vi "traj_generator.vi"(0 "v_max":dbl, 1 "a_max":dbl, 2 "p_i":dbl, 3 "p_f":dbl, 4 "v_i":dbl, 5 "v_f":dbl, 6 "trigger":bool, 7 "t":dbl) -> (14 "p":dbl format="%0.2f", 15 "v":dbl format="%0.2f", 16 "a":dbl)   [LabVIEW 2012]
doc: "Based on :\nTime-Optimal Online Trajectory Generator for Robotic Manipulators \nFransisco Ramos. et al.\n\nInputs:\na_max = maximum admissible acceleration\nv_max = maximum admissible speed\np_i = current position\np_f = target position\nv_i = current velocity\nv_f = target velocity\ntrigger = tell the algorithm to proceed\nThe trigger signal is a transition from 0 to 1 (edge triggered)\n\nOutputs:\na = acceleration trajectory\nv = velocitiy trajectory\np = position trajectory"
panel:
  out "is_triggered":bool
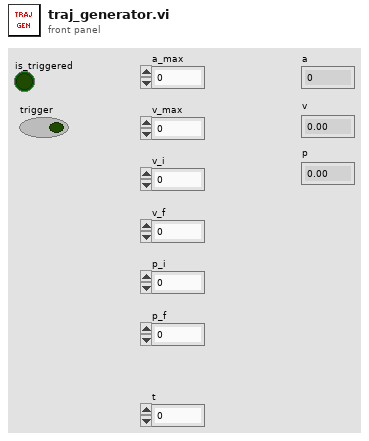
[diagram p1: front panel]
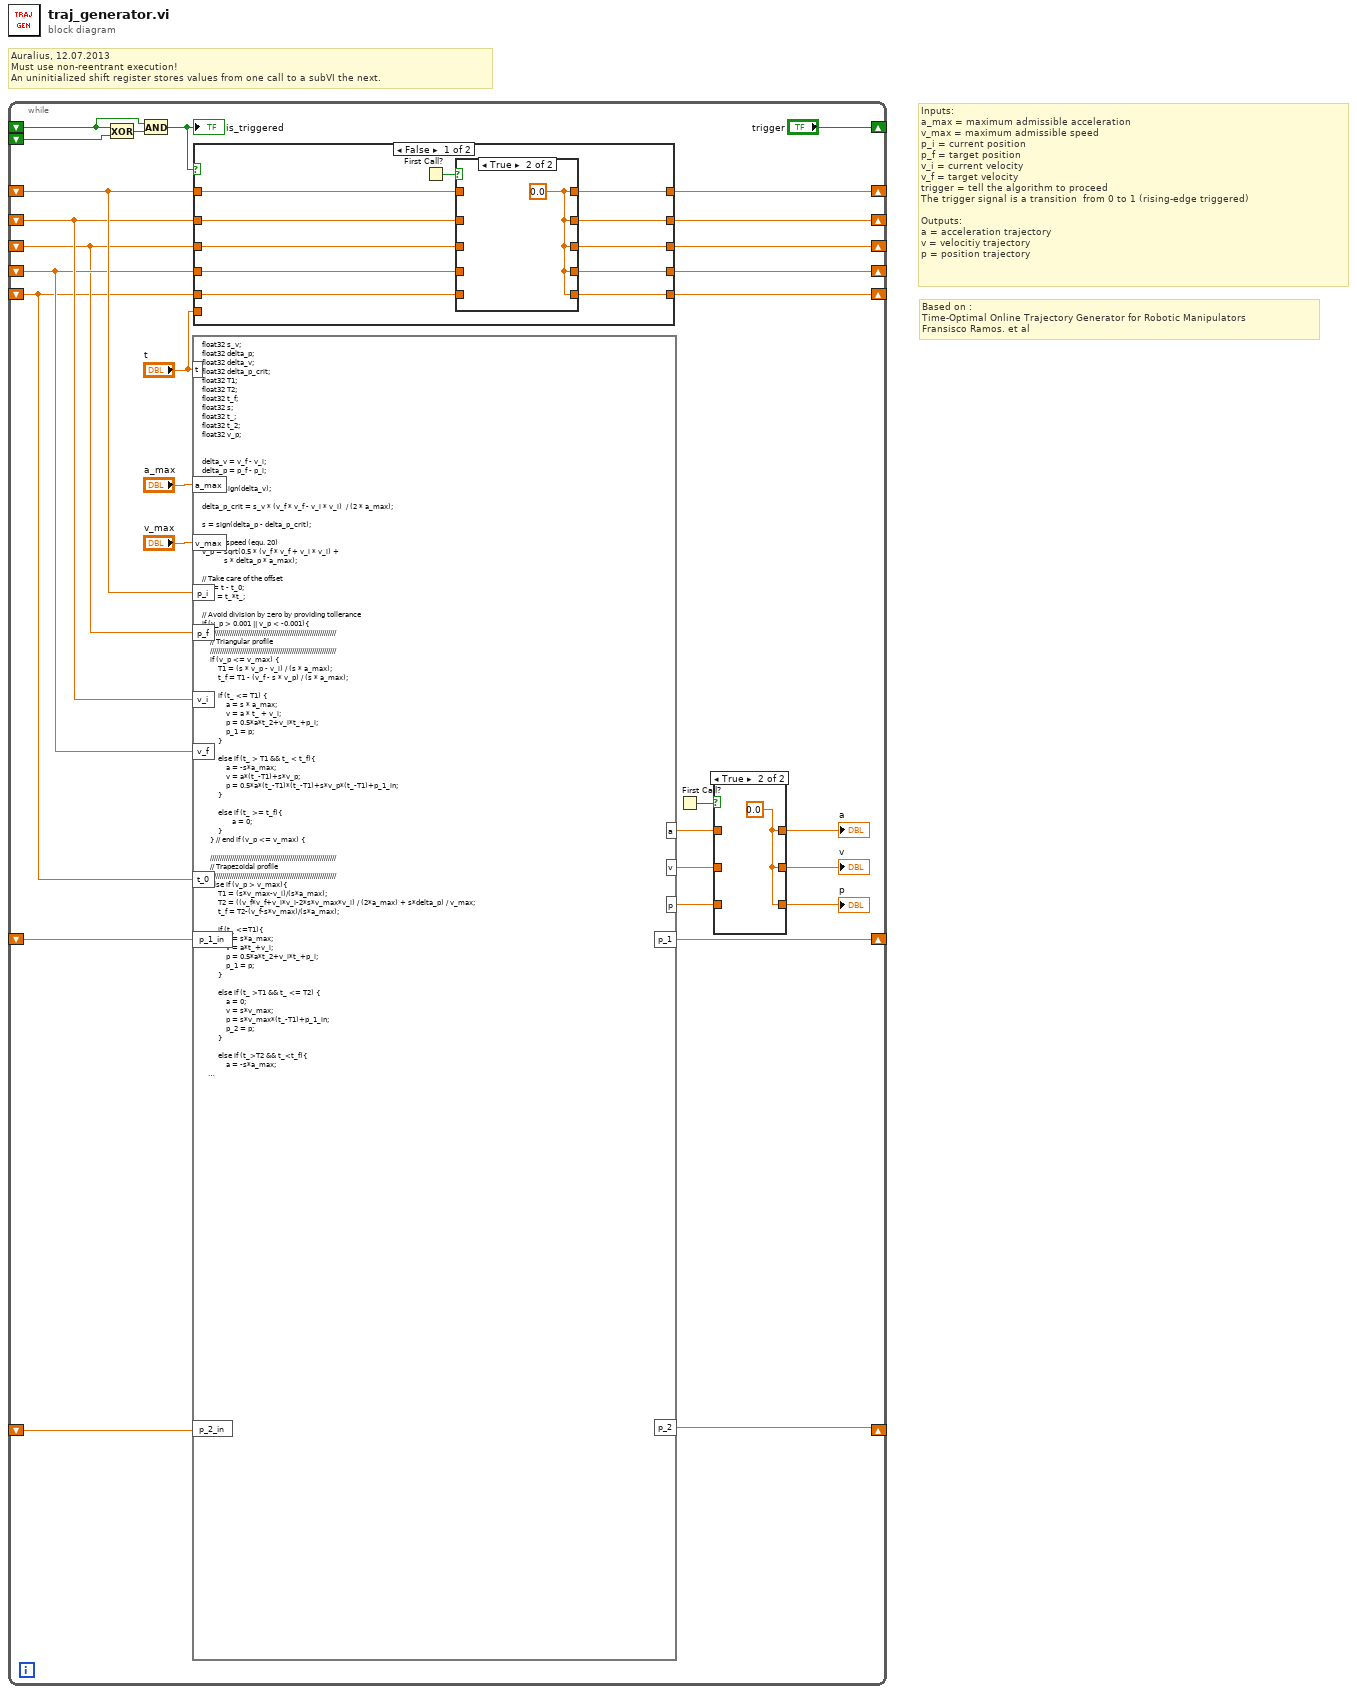
[diagram p0: block diagram]
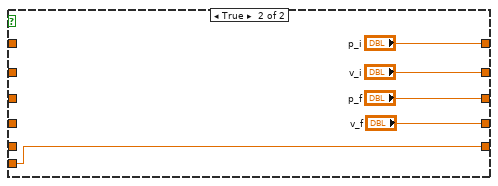
[diagram p4: hidden frame]
diagram:
  # "Based on :\nTime-Optimal Online Trajectory Generator for Robotic Manipulators \nFransisco Ramos. et al"
  # "Inputs:\na_max = maximum admissible acceleration\nv_max = maximum admissible speed\np_i = current position\np_f = target position\nv_i = current velocity\nv_f = target velocity\ntrigger = tell the algorithm to proceed\nThe trigger signal is a transition  from 0 to 1 (rising-edge triggered)\n\nOutputs:\na = acceleration trajectory\nv = velocitiy trajectory\np = position trajectory"
  # "Auralius, 12.07.2013\nMust use non-reentrant execution!\nAn uninitialized shift register stores values from one call to a subVI the next."
  n1 = while {
    shift-right: ["trigger"] -> _
    shift-left: _ -> [w25]
    shift-left: _ -> [w26]
    shift-right: [w23] -> _
    shift-left: _ -> [w21]
    shift-right: [w22] -> _
    shift-left: _ -> [w20]
    shift-right: [w18] -> _
    shift-left: _ -> [w15]
    shift-right: [w17] -> _
    shift-left: _ -> [w16]
    shift-right: [w14] -> _
    shift-left: _ -> [w13]
    shift-right: [w9] -> _
    shift-left: _ -> [w10]
    shift-right: [w8] -> _
    shift-left: _ -> [w7]
    stop <- FALSE continue-if-true
    n2 = Exclusive Or(1:w26, 2:w25) -> (0:w24:bool)
    n3 = And(x=w25, y=w24) -> (x .and. y?=w1:bool)
    "is_triggered" <- w1
    n4 = formula code="float32 s_v;\nfloat32 delta_p;\nfloat32 delta_v;\nfloat32 delta_p_crit;\nfloat32 T1;\nfloat32 T2;\nfloat32 t_f;\nfloat32 s;\nfloat32 t_;\nfloat32 t_2;\nfloat32 v_p;\n\n\ndelta_v = v_f - v_i;\ndelta_p = p_f - p_i;\n\ns_v = sign(delta_v);\n\ndelta_p_crit = s_v * (v_f * v_f - v_i * v_i)  / (2 * a_max);\n\ns = sign(delta_p - delta_p_crit);\n\n// Peak speed (equ. 20)\nv_p = sqrt(0.5 * (v_f * v_f + v_i * v_i) + \n           s * delta_p * a_max);\n\n// Take care of the offset\n t_ = t - t_0;\n t_2 = t_*t_;\n\n// Avoid division by zero by providing tollerance          \nif (v_p > 0.001 || v_p < -0.001){\n    ///////////////////////////////////////////////////////////////\n    // Triangular profile\n    ///////////////////////////////////////////////////////////////\n    if (v_p <= v_max) {\n        T1 = (s * v_p - v_i) / (s * a_max);\n        t_f = T1 - (v_f - s * v_p) / (s * a_max);\n\n        if (t_ <= T1) {\n            a = s * a_max;\n            v = a * t_ + v_i;\n            p = 0.5*a*t_2+v_i*t_+p_i;\n            p_1 = p;\n        } \n\n        else if (t_ > T1 && t_ < t_f){\n            a = -s*a_max;\n            v = a*(t_-T1)+s*v_p;\n            p = 0.5*a*(t_-T1)*(t_-T1)+s*v_p*(t_-T1)+p_1_in;\n        }\n\n        else if (t_ >= t_f){\n               a = 0;\n        }\n    } // end if (v_p <= v_max) {\n\n    ///////////////////////////////////////////////////////////////\n    // Trapezoidal profile\n    ///////////////////////////////////////////////////////////////\n    else if (v_p > v_max){\n        T1 = (s*v_max-v_i)/(s*a_max);\n        T2 = ((v_f*v_f+v_i*v_i-2*s*v_max*v_i) / (2*a_max) + s*delta_p) / v_max;\n        t_f = T2-(v_f-s*v_max)/(s*a_max);\n\n        if (t_ <=T1){\n            a = s*a_max;\n            v = a*t_+v_i;\n            p = 0.5*a*t_2+v_i*t_+p_i; \n            p_1 = p;\n        }\n         \n        else if (t_ >T1 && t_ <= T2) {\n            a = 0;\n            v = s*v_max;\n            p = s*v_max*(t_-T1)+p_1_in;\n            p_2 = p;\n        }\n        \n        else if (t_>T2 && t_<t_f){\n            a = -s*a_max;\n            v = a*(t_-T2)+s*v_max;\n            p = 0.5*a*(t_-T2)*(t_-T2)+s*v_max*(t_-T2)+p_2_in;\n        }\n\n        else if (t_ >= t_f){\n               a = 0;\n        }\n    } // end else if (v_p > v_max){\n} \n\nelse{\n    a=0;\n    v=v_i;\n    p = p_i;\n}  \n///////////////////////////////////////////////////////////////"("a_max"="a_max", "v_max"="v_max", "v_i"=w20, "v_f"=w16, "p_i"=w21, "p_f"=w15, "t"="t", "t_0"=w13, "p_1_in"=w10, "p_2_in"=w7) -> ("a"=w19:dbl, "v"=w12:dbl, "p"=w11:dbl, "p_1"=w9:dbl, "p_2"=w8:dbl)
    n5 = case shown="False" w1 {
      tunnel: [w36 "p_i"] -> w23
      tunnel: [w38 "v_i"] -> w22
      tunnel: w21 -> [w35 _]
      tunnel: w20 -> [w37 _]
      tunnel: [w40 "p_f"] -> w18
      tunnel: [w42 "v_f"] -> w17
      tunnel: w15 -> [w39 _]
      tunnel: w16 -> [w41 _]
      tunnel: [w44 w52] -> w14
      tunnel: w13 -> [w43 _]
      tunnel: "t" -> [_ w52]
      frame False {
        n6 = First Call?() -> (First Call?: T/F=w45:bool)
        n7 = case shown="True" w45 {
          tunnel: [w50 w51] -> w44
          tunnel: w43 -> [w50 _]
          tunnel: [w49 w51] -> w42
          tunnel: w41 -> [w49 _]
          tunnel: [w48 w51] -> w40
          tunnel: w39 -> [w48 _]
          tunnel: [w47 w51] -> w38
          tunnel: w37 -> [w47 _]
          tunnel: [w46 w51] -> w36
          tunnel: w35 -> [w46 _]
          frame False {
          }
          frame True {
            w51 = 0.0 ("p_i")
          }
        }
      }
      frame True {
      }
    }
    n8 = First Call?() -> (First Call?: T/F=w5:bool)
    n9 = case shown="True" w5 {
      tunnel: w19 -> [w33 _]
      tunnel: w12 -> [w32 _]
      tunnel: w11 -> [w31 _]
      tunnel: [w33 w34] -> w4
      tunnel: [w32 w34] -> w3
      tunnel: [w31 w34] -> w2
      frame False {
      }
      frame True {
        w34 = 0.0 ("a")
      }
    }
    "a" <- w4
    "v" <- w3
    "p" <- w2
  }
